vi "ConfigureRF.vi"(8 "error in (no error)":errorcluster, 11 "reference in":refnum<class "niMmWave_Transceiver.lvclass">) -> (0 "error out":errorcluster, 3 "reference out":refnum<class "niMmWave_Transceiver.lvclass">)   [LabVIEW 2019, in "niMmWave_Transceiver.lvclass"]
doc: "Configures RF setting at specified port:\n<b>Frequency</b> - operating frequency (RF/IF)\n<b>Gain</b> - Signal gain"
uses:
  niMmWave_Transceiver.lvclass
  C:/Barkhausen mmWave radar/Development/modules/mmw_instrument/src_LabVIEW/Host/SubVIs/mmWave instrument_class/mmWave instrument.lvclass
  Low-level/TypeDefs/Front End Configuration.ctl
  Low-level/TypeDefs/Channel Configuration.ctl
  <instrlib>/niMmWave/ni3620/Config/v1/Host/Public/Typedefs/mmWave Port.ctl
  mmWave instrument_class/mmWave instrument.lvclass
  mmWave HW Control/mmWave HW Control.lvlib
  <instrlib>/niMmWave/ni3620/Config/v1/Host/niMmWave Config v1 Host.lvlib
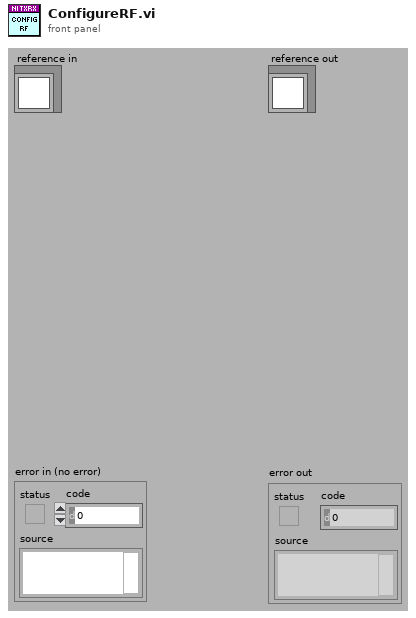
[diagram p1: front panel]
types:
  T1 = typedef "niMmWave Config v1 Host.lvlib/mmWave Port.ctl" = string
  T2 = typedef "Front End Configuration.ctl" = cluster{"port select":enum16{"IF Port", "Loopback", "Sync Port"}, "Rx hardware configuration":T3, "Tx hardware configuration":T3}
  T3 = typedef "Channel Configuration.ctl" = cluster{"gain (dB)":dbl, "frequency (Hz)":dbl, "mmWave adapter":string, "adapter active port":T1}
  T4 = typedef "niMmWave_Transceiver.lvclass/ObjectAttributesRef.ctl" = refnum<data-value>
  T5 = typedef "mmWave instrument.lvclass/ObjectAttributes.ctl" = cluster{"mode":T6, "instr state":T7, "Max Fs":dbl, "Equalization coeff":cdb[], "LO sync en":bool, "Trig sync en":bool, "LO sources":T8, "LO Export":T9, "Fc.range":cluster{"min":dbl, "max":dbl}, "Sync mode":T10, "equalization en":bool, "sequence":string[]}
  T6 = typedef "mmWave instrument.lvclass/Instrument mode.ctl" = enum16{"RF", "IF", "BB"}
  T7 = typedef "mmWave instrument.lvclass/Instrument state.ctl" = enum16{"Off", "Initialization", "Configuration", "Running", "Calibration"}
  T8 = typedef "mmWave HW Control.lvlib/LO sources.ctl" = cluster{"RX/LO1 src":string, "TX/LO1 src":string, "LO2 src":string}
  T9 = typedef "mmWave HW Control.lvlib/LO export.ctl" = cluster{"TX LO1 export":bool, "TX LO1 export level":dbl, "RX LO1 export":bool, "RX LO1 export level":dbl, "LO2 export":bool, "LO2 export level":dbl}
  T10 = typedef "mmWave instrument.lvclass/Sync mode.ctl" = enum16{"Slave", "Master"}
  T11 = typedef "niMmWave_Transceiver.lvclass/ObjectAttributes.ctl" = cluster{"session":T12[], "HW.RX resources":T26, "RF config":T27, "RX trigger options":T28, "TX trigger options":T28, "RX samples":i32, "Downloaded Bursts":map{string, T31}, "TX Fs":dbl, "RX Fs":dbl, "burst sequence":string[]}
  T12 = typedef "Session.ctl" = cluster{"3620 session":refnum<queue>, "tx baseband session":T13, "rx baseband session":T21, "tx gain (dB)":dbl, "rx gain (dB)":dbl, "hardware configuration":T22, "gain ranging":T24[], "pxi trigger bus information":T25}
  T13 = typedef "Tx Baseband Session.ctl" = cluster{"3610 session":T14, "7902 reference":T20}
  T14 = typedef "ni3610_and_ni3630_Driver_Lib.lvlib/Main Settings.ctl" = cluster{"VISA resource name":refnum<visa-resource-name>, "Address Space":T15, "window_offset":u32, "register_addresses":T16, "required_MM_fpga_version":cluster{"signature":u32, "hardware":u32, "current revision":u32, "oldest revision":u32}, "CPLD Oldest Compat Version ":cluster{"hardware":u32, "CPLD firmware":u32}, "MM_FPGA_image_location":string, "is_init":bool, "card_type":T17, "DacLmkConfigFileName":string, "AdcLmkConfigFileName":string, "AdcConfigFileName":string, "DacConfigFileName_RevA":string, "DacConfigFileName_RevB":string, "Mulde hardware revision":u8, "bypass DAC PLL\n":bool, "IQ Card Revision":T18, "board capability":T19}
  T15 = typedef "VISA Register Access Address Space.ctl" = u16
  T16 = typedef "ni3610_and_ni3630_Driver_Lib.lvlib/Register Adresses.ctl" = cluster{"MM based Registers":cluster{"Revision":u32, "OldestCompatRev":u32, "signature":u32, "scratch":u32, "LedControl":u32, "BoardHwRev":u32, "BoardControl":u32, "ThermalStatus":u32, "BasebandStatus":u32, "BasebandControl":u32, "BasebandAuxSetup":u32, "BasebandAuxStatus":u32, "LmkSyncOutSetup":u32, " AdcSyncOutSetup":u32, " InjSyncOutSetup":u32, " PxiTrig0OutSetup":u32, " PxiTrig1OutSetup":u32, " PxiTrig2OutSetup":u32, " PxiTrig3OutSetup":u32, " PxiTrig4OutSetup":u32, " PxiTrig5OutSetup":u32, " PxiTrig6OutSetup":u32, " PxiTrig7OutSetup":u32}, "CPLD based Registers":cluster{"SlaveSignature":u32, "SlaveRevision":u32, "SlaveOldestCompatRev":u32, "SlaveScratch":u32, "SlaveSetup":u32, "SlaveStatus":u32, "IDacReg_offset":u32, "LMKRegGrp0_offset":u32, "QDacReg_offset":u32, "BrdTempSensorVal":u32, "TempSensorPowerDown":u32, "GPIOReg_offset":u32, "IAdcReg_offset":u32, "QAdcReg_offset":u32, "LMKRegGrp1_offset":u32, "QadcTempSensorVal":u32, "IadcTempSensorVal":u32, "RevisionReg":u32, "VcxoReg":u32, "CpldStatusReg":u32, "PowerReg":u32, "VBiasEnReg":u32, "ExtRefOeReg":u32, "QdacCtrlReg":u32, "QdacStatusReg":u32, "IdacCtrlReg":u32, "IdacStatusReg":u32, "QdacJtagIn":u32, "QdacJtagOut":u32, "IdacJtagIn":u32, "IdacJtagOut":u32, "IqDcSetupReg":u32, "QadcStatusReg":u32, "IadcStatusReg":u32, "BrdSetupReg":u32, "IqDcRevisionReg":u32, "PllStatusReg":u32, "EndpointScratchReg":u32, "AdcSyncCfgReg":u32, "IqCardOpampReg":u32}, "CPLD Register Offset":u32, "MM  Register Offset":u32, " PxiTrig0OutSetup":u32}
  T17 = typedef "ni3610_and_ni3630_Driver_Lib.lvlib/Base Card Type.ctl" = enum16{"unspecified", "ADC", "DAC"}
  T18 = typedef "ni3610_and_ni3630_Driver_Lib.lvlib/IQ Card Revision.ctl" = enum16{"RevA", "RevB", "RevC", "RevD"}
  T19 = typedef "ni3610_and_ni3630_Driver_Lib.lvlib/Board Capability.ctl" = cluster{"baseband sync":enum16{"no baseband sync", "baseband sync"}}
  T20 = typedef "Blank FPGA Reference.ctl" = refnum<k20>
  T21 = typedef "Rx Baseband Session.ctl" = cluster{"3630 session":T14, "7902 reference":T20}
  T22 = typedef "Hardware Configuration.ctl" = cluster{"direction":T23, "baseband only":bool}
  T23 = typedef "Direction.ctl" = enum16{"Transceiver", "Receiver", "Transmitter"}
  T24 = typedef "Gain Ranging.ctl" = cluster{"gain ranging active scope":string, "gain ranging stream session":refnum<k20>}
  T25 = typedef "PXI Trigger Bus Info.ctl" = cluster{"chassis resource name":refnum<visa-resource-name>, "7902R (TX)":i16, "3610 (TX)":i16, "3620 (IF)":i16, "3630 (RX)":i16, "7902R (RX)":i16}
  T26 = typedef "mmWave HW Control.lvlib/HW TXRX resources cluster.ctl" = cluster{"TX_DAC":refnum<visa-resource-name>, "TX_FPGA":tag, "IF":tag, "RX_ADC":refnum<visa-resource-name>, "RX_FPGA":tag}
  T27 = typedef "mmWave HW Control.lvlib/HW TXRX RF config cluster.ctl" = cluster{"TX.Frequency":dbl, "TX.Gain":dbl, "TX.mmWave adapter":string, "RX.Frequency":dbl, "RX.Gain":dbl, "RX.mmWave adapter":string}
  T28 = typedef "TX trigger config.ctl" = cluster{"delay":dbl, "trig source":T29, "PXI src":i32, "export":T30, "PXI dest":i32}
  T29 = typedef "FPGA Utility.lvlib/FPGA driver trigger source.ctl" = enum16{"Use Tclk", "PXI_Trig", "Aurora RX trig"}
  T30 = typedef "FPGA Utility.lvlib/FPGA driver trigger destination.ctl" = enum16{"None", "Source trig", "Synced trig", "Delayed sync"}
  T31 = typedef "niMmWave_Transceiver.lvclass/BurstInfo.ctl" = cluster{"starting addr":u32, "end addr":u32}
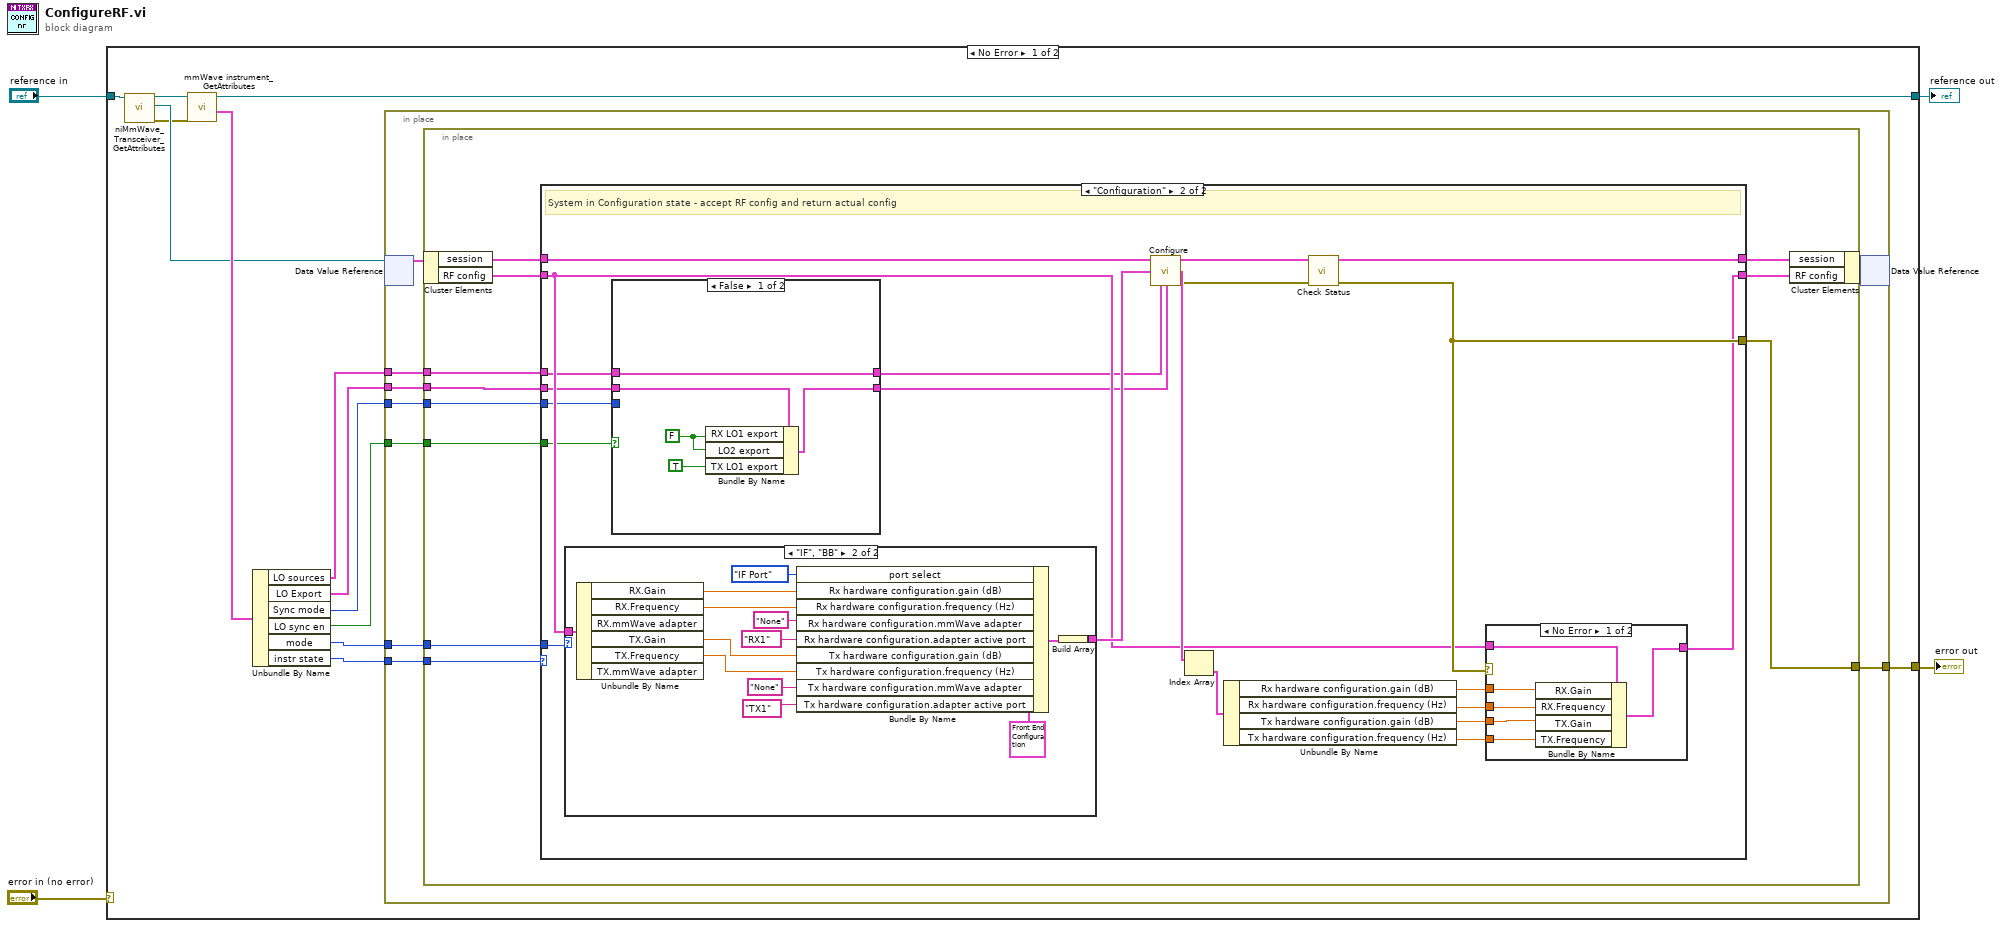
[diagram p0: block diagram]
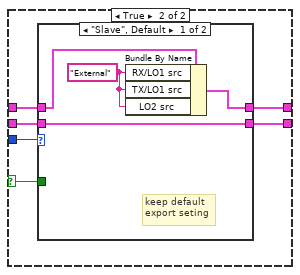
[diagram p3: hidden frame]
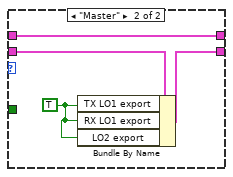
[diagram p4: hidden frame]
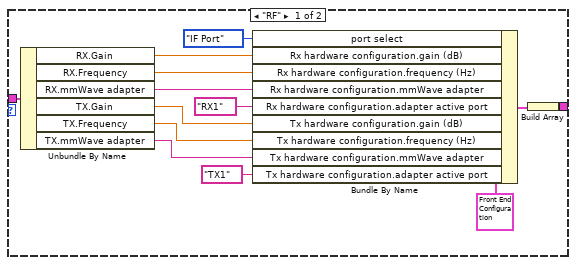
[diagram p6: hidden frame]
diagram:
  n1 = case shown="No Error" "error in (no error)" {
    selector: "error in (no error)" -> [_ w114]
    tunnel: [w11 w114] -> w3
    tunnel: [w15 w113] -> w1
    tunnel: "reference in" -> [w16 w113]
    frame No Error {
      n2 = call "niMmWave_Transceiver_GetAttributes.vi"("reference in"=w16) -> ("error out"=w12:errorcluster, "attributes ref"=w13:T4, "reference out"=w17:refnum<class "niMmWave_Transceiver.lvclass">)  [unwired: 7 in, 1 out]
      n3 = call "mmWave instrument_GetAttributes.vi"("error in (no error)"=w12, "reference in"=w17) -> ("attributes"=w14:T5, "reference out"=w15:refnum<class "niMmWave_Transceiver.lvclass">)  [unwired: 6 in, 2 out]
      n4 = Unbundle By Name(w14) -> ("LO sources"=w7:T8, "LO Export"=w6:T9, "Sync mode"=w5:T10, "LO sync en"=w8:bool, "mode"=w10:T6, "instr state"=w9:T7)
      n5 = in-place {
        in-place-border: [w24] -> w11
        in-place-border: w10 -> [w23]
        in-place-border: w9 -> [w22]
        in-place-border: w8 -> [w21]
        in-place-border: w7 -> [w20]
        in-place-border: w6 -> [w19]
        in-place-border: w5 -> [w18]
        n6 = in-place-dvr #1(w13) -> (w26:T11)  [unwired: 1 out]
        n7 = in-place {
          in-place-border: [w34] -> w24
          in-place-border: w23 -> [w35]
          in-place-border: w22 -> [w32]
          in-place-border: w21 -> [w30]
          in-place-border: w20 -> [w29]
          in-place-border: w19 -> [w28]
          in-place-border: w18 -> [w27]
          n8 = in-place-cluster #2(w26) -> ("session"=w37:T12[], "RF config"=w31:T27)
          n9 = case shown="\"Configuration\"" w32 {
            tunnel: w37 -> [w39 w58]
            tunnel: [w39 w57] -> w36
            tunnel: w35 -> [_ w56]
            tunnel: [_ w52] -> w34
            tunnel: [w38 w47] -> w33
            tunnel: w31 -> [w38 w46]
            tunnel: w30 -> [_ w45]
            tunnel: w29 -> [_ w44]
            tunnel: w28 -> [_ w43]
            tunnel: w27 -> [_ w40]
            frame "Off", Default {
            }
            frame "Configuration" {
              # "System in Configuration state - accept RF config and return actual config"
              n10 = case shown="\"IF\", \"BB\"" w56 {
                tunnel: [w99 w112] -> w59
                tunnel: w46 -> [w93 w107]
                frame "RF" {
                  n11 = Unbundle By Name(w93) -> ("RX.Gain"=w92:dbl, "RX.Frequency"=w91:dbl, "RX.mmWave adapter"=w90:string, "TX.Gain"=w89:dbl, "TX.Frequency"=w88:dbl, "TX.mmWave adapter"=w87:string)
                  n12 = Bundle By Name(cluster=T2 {"port select"=enum."Loopback", "Rx hardware configuration"={"gain (dB)"=15.0, "frequency (Hz)"=12000000000.0, "mmWave adapter"="None", "adapter active port"=""}, "Tx hardware configuration"={"gain (dB)"=-15.0, "frequency (Hz)"=12000000000.0, "mmWave adapter"="None", "adapter active port"=""}} ("device configuration [channel]"), "port select"=enum16{"IF Port", "Loopback", "Sync Port"}."IF Port", "Rx hardware configuration.gain (dB)"=w92, "Rx hardware configuration.frequency (Hz)"=w91, "Rx hardware configuration.mmWave adapter"=w90, "Rx hardware configuration.adapter active port"=T1 "RX1", "Tx hardware configuration.gain (dB)"=w89, "Tx hardware configuration.frequency (Hz)"=w88, "Tx hardware configuration.mmWave adapter"=w87, "Tx hardware configuration.adapter active port"=T1 "TX1") -> (w98:T2)
                  n13 = Build Array(w98) -> (w99:T2[])
                }
                frame "IF", "BB" {
                  n14 = Unbundle By Name(w107) -> ("RX.Gain"=w106:dbl, "RX.Frequency"=w105:dbl, "TX.Gain"=w104:dbl, "TX.Frequency"=w103:dbl)  [unwired: 2 out]
                  n15 = Bundle By Name(cluster=T2 {"port select"=enum."Loopback", "Rx hardware configuration"={"gain (dB)"=15.0, "frequency (Hz)"=12000000000.0, "mmWave adapter"="None", "adapter active port"=""}, "Tx hardware configuration"={"gain (dB)"=-15.0, "frequency (Hz)"=12000000000.0, "mmWave adapter"="None", "adapter active port"=""}} ("device configuration [channel]"), "port select"=enum16{"IF Port", "Loopback", "Sync Port"}."IF Port", "Rx hardware configuration.gain (dB)"=w106, "Rx hardware configuration.frequency (Hz)"=w105, "Rx hardware configuration.mmWave adapter"="None", "Rx hardware configuration.adapter active port"=T1 "RX1", "Tx hardware configuration.gain (dB)"=w104, "Tx hardware configuration.frequency (Hz)"=w103, "Tx hardware configuration.mmWave adapter"="None" ("Rx hardware configuration.mmWave adapter"), "Tx hardware configuration.adapter active port"=T1 "TX1") -> (w111:T2)
                  n16 = Build Array(w111) -> (w112:T2[])
                }
              }
              n17 = case shown="False" w45 {
                selector: w45 -> [_ w66]
                tunnel: w44 -> [w65 w67]
                tunnel: w43 -> [w64 w71]
                tunnel: [w65 w68] -> w42
                tunnel: [w63 w70] -> w41
                tunnel: w40 -> [_ w69]
                frame False {
                  w62 = FALSE
                  n18 = Bundle By Name(cluster=w64, "RX LO1 export"=w62, "LO2 export"=w62, "TX LO1 export"=TRUE) -> (w63:T9)
                }
                frame True {
                  n19 = case shown="\"Slave\", Default" w69 {
                    tunnel: w71 -> [w72 w79]
                    tunnel: [w72 w78] -> w70
                    tunnel: [w74 w76] -> w68
                    tunnel: w67 -> [w75 w76]
                    tunnel: w66 -> [_ _]
                    frame "Slave", Default {
                      w73 = "External" ("RX/LO1 src")
                      # "keep default\nexport seting"
                      n20 = Bundle By Name(cluster=w75, "RX/LO1 src"=w73, "TX/LO1 src"=w73, "LO2 src"=w73) -> (w74:T8)
                    }
                    frame "Master" {
                      w77 = TRUE
                      n21 = Bundle By Name(cluster=w79, "TX LO1 export"=w77, "RX LO1 export"=w77, "LO2 export"=w77) -> (w78:T9)
                    }
                  }
                }
              }
              n22 = call "Configure.vi"("session in"=w58, "device configuration [channel]"=w59, "LO sources"=w42, "LO Export"=w41) -> ("session out"=w60:T12[], "coerced device configuration [channel]"=w55:T2[], "error out"=w53:errorcluster)  [unwired: 9 in]
              n23 = Index Array(array=w55) -> (element=w54:T2)  [unwired: 1 in]
              n24 = Unbundle By Name(w54) -> ("Rx hardware configuration.gain (dB)"=w51:dbl, "Rx hardware configuration.frequency (Hz)"=w50:dbl, "Tx hardware configuration.gain (dB)"=w49:dbl, "Tx hardware configuration.frequency (Hz)"=w48:dbl)
              n25 = call "Check Status.vi"("session in"=w60, "error in"=w53) -> ("session out"=w57:T12[], "error out"=w52:errorcluster)  [unwired: 9 in, 3 out]
              n26 = case shown="No Error" w52 {
                tunnel: w46 -> [w85 w86]
                tunnel: w51 -> [w80 _]
                tunnel: w50 -> [w81 _]
                tunnel: w49 -> [w83 _]
                tunnel: w48 -> [w82 _]
                tunnel: [w84 w86] -> w47
                frame No Error {
                  n27 = Bundle By Name(cluster=w85, "RX.Gain"=w80, "RX.Frequency"=w81, "TX.Gain"=w83, "TX.Frequency"=w82) -> (w84:T27)
                }
                frame Error {
                }
              }
            }
          }
          n28 = in-place-cluster #2("session"=w36, "RF config"=w33) -> (w25:T11)
        }
        n29 = in-place-dvr #1(w25) -> ()  [unwired: 2 out]
      }
    }
    frame Error {
    }
  }
  "error out" <- w3
  "reference out" <- w1
